vi "Untitled 1.vi"() -> ()   [LabVIEW 2016]
panel:
  in  "Start":bool
  in  "ShooterState":enum16{"Idle", "Recover", "Shoot", "QueFuel"}(ring)
  in  "Shoot Command":bool
  in  "Turret Aimed":bool
  in  "Shooter Motor Speed Good":bool
  in  "Ball In Position":bool
  in  "Turret Aimed":bool
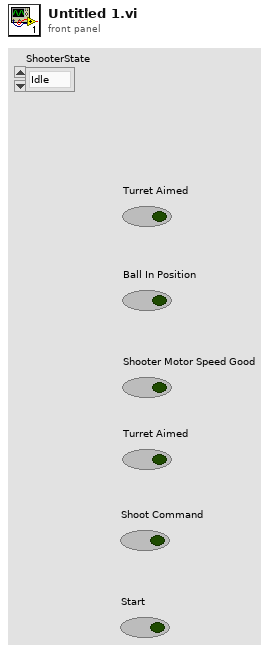
[diagram p1: front panel]
types:
  T1 = enum16{"Idle", "BottomFeeder", "TurretMotor", "ShooterMotor/TopFeederON", "TopFeederON"}
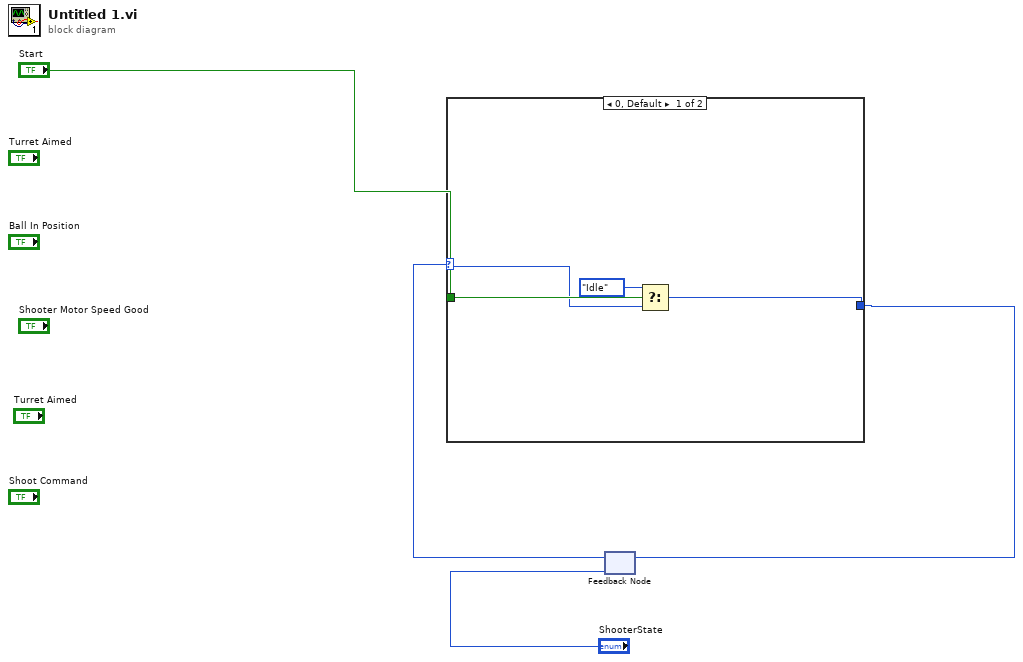
[diagram p0: block diagram]
diagram:
  n1 = feedback #1("ShooterState") -> (w3:u16)
  n2 = case shown="0, Default" w3 {
    selector: w3 -> [w7 _]
    tunnel: [w6 _] -> w2
    tunnel: "Start" -> [w8 _]
    frame 0, Default {
      n3 = Select(t=T1."Idle", s=w8, f=w7) -> (s? t:f=w6:u16)
    }
    frame 0 {
    }
  }
  n4 = feedback-in #1(w2) -> ()
